vi "scan lines, output data.vi"(9 "width":i32, 10 "no. of scanning lines":i32, 11 "Refnum in":T1) -> (1 "std dev arrays":sgl[](array[numeric]), 2 "mean Array":sgl[](array[numeric]), 3 "Refnum out":T1)   [LabVIEW 2011]
uses:
  <vilib>/vision/Image Controls.llb/IMAQ Image.ctl
  <vilib>/vision/NI_Vision_Development_Module.lvlib
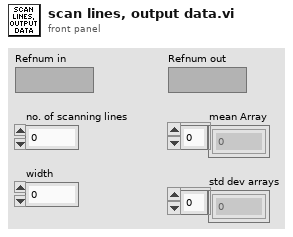
[diagram p1: front panel]
types:
  T1 = typedef "IMAQ Image.ctl" = refnum<image>
  T2 = typedef "ROI Descriptor" = cluster{"Global Rectangle":i32[], "Contours":cluster{"ID":enum32{"External", "Internal"}, "Type":u32, "Coordinates":i32[]}[]}
  T3 = cluster{"Min":sgl, "Max":sgl, "Mean":sgl, "Std Dev":sgl, "Count":i32}
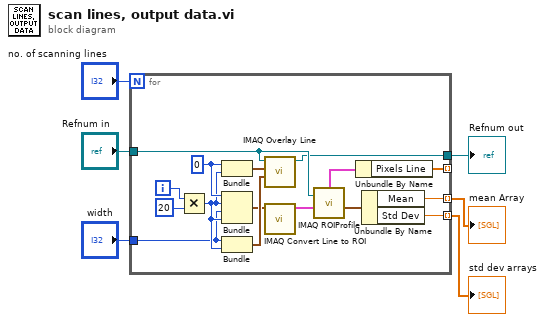
[diagram p0: block diagram]
diagram:
  n1 = for {
    N: "no. of scanning lines" -> [_]
    tunnel: "Refnum in" -> [w13]
    tunnel: [w12] -> _ mode=indexing
    tunnel: [w9] -> w4 mode=indexing
    tunnel: [w10] -> w1
    tunnel: [w8] -> w3 mode=indexing
    tunnel: "width" -> [w7]
    i -> [w18]
    w19 = 0 ("End Y")
    n2 = Multiply(x=w18, y=20) -> (x*y=w15:i32)
    n3 = Bundle("End Y"=w19, w15) -> (w22:cluster{"End Y":i32, i32})  [unwired: 1 in]
    n4 = Bundle("End Y"=w19, w15, "width"=w7, w15) -> (w17:cluster{"End Y":i32, i32, "width":i32, i32})  [unwired: 1 in]
    n5 = Bundle("width"=w7, w15) -> (w21:cluster{"width":i32, i32})  [unwired: 1 in]
    n6 = call "IMAQ Overlay Line"("End Point"=w21, "Start Point"=w22, "Image"=w13) -> ("Image Out"=w10:T1)  [unwired: 7 in, 1 out]
    n7 = call "IMAQ Convert Line to ROI"("Line"=w17) -> ("ROI Descriptor"=w16:T2)  [unwired: 8 in, 1 out]
    n8 = call "IMAQ ROIProfile"("ROI Descriptor"=w16, "Image"=w13) -> ("ROI Pixel Statistics"=w11:T3, "ROI Graph"=w20:cluster{"x0":sgl, "dx":sgl, "Pixels Line":sgl[]})  [unwired: 2 in, 3 out]
    n9 = Unbundle By Name(w20) -> ("Pixels Line"=w12:sgl[])
    n10 = Unbundle By Name(w11) -> ("Mean"=w9:sgl, "Std Dev"=w8:sgl)
  }
  "mean Array" <- w4
  "std dev arrays" <- w3
  "Refnum out" <- w1
